vi "Return Data Packet.vi"(7 "Connection ID":string, 8 "error in (no error)":errorcluster, 9 "Packet Data":variant, 10 "Packet Header":string, 11 "IPacketReturn in":refnum<class "EventMessageRxCallback.lvclass">) -> (0 "error out":errorcluster)   [LabVIEW 2020, in "EventMessageRxCallback.lvclass"]
uses:
  <vilib>/gpm_packages/@cs/Network-interface/Examples/EventMessageRxCallback/EventMessageRxCallback.lvclass
  <vilib>/gpm_packages/@cs/Network-interface/Examples/EventMessageRxCallback/EventMessageRxCallback.lvclass/EventMessageRxCallback.ctl
  <vilib>/gpm_packages/@cs/Network-interface/Examples/EventMessageRxCallback/Message Information Type.ctl
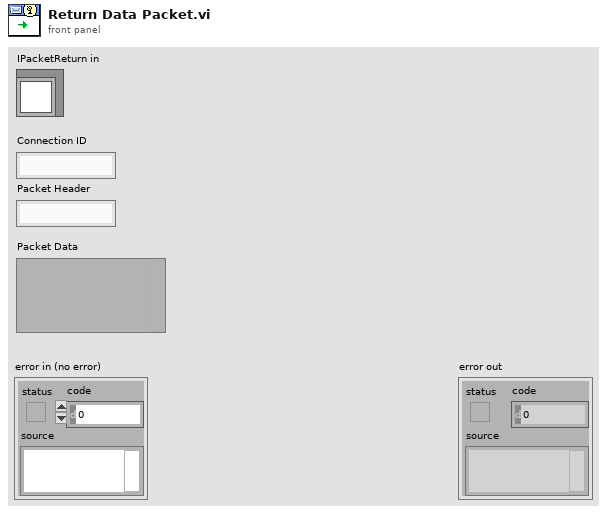
[diagram p1: front panel]
types:
  T1 = typedef "EventMessageRxCallback.lvclass/Message Information Type.ctl" = cluster{"Connection ID":string, "Message":string, "Data":variant}
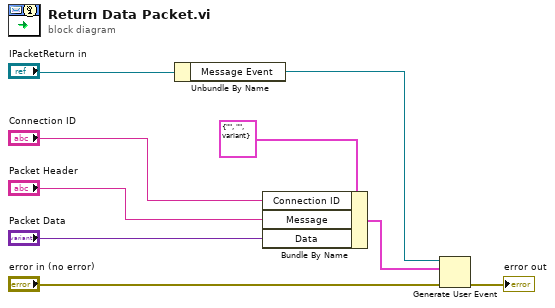
[diagram p0: block diagram]
diagram:
  n1 = Unbundle By Name("IPacketReturn in") -> ("Message Event"=w1:refnum<user-event>)
  n2 = Bundle By Name(cluster=T1 {"Connection ID"="", "Message"="", "Data"=variant} ("Message Information"), "Connection ID"="Connection ID", "Message"="Packet Header", "Data"="Packet Data") -> (w3:T1)
  n3 = Generate User Event(user event=w1, event data cluster=w3, error in="error in (no error)") -> (error out=→"error out":errorcluster)  [unwired: 1 in, 1 out]
